vi "Import File - Tx XML.vi"(6 "Root Node":refnum<k24>, 8 "error in (no error)":errorcluster) -> (0 "error out":errorcluster, 5 "Tx Packets":T1 {"Tx Packet Data"."threadOptions"."pclDecimation" max=16 step=1; "Tx Packet Data"."threadOptions"."loopPeriod" max=16 step=1; "Tx Packet Data"."threadOptions"."targetPriority" min=-2 max=16 step=1; "Tx Packet Data"."threadOptions"."targetProcessor" min=-2 max=16 step=1; "Tx Packet Data"."Endianness" items=["big-endian"=0, "little-endian"=2]})   [LabVIEW 2019, in "UDP-Custom-Device System Explorer.lvlib"]
uses:
  UDP-Custom-Device System Explorer.lvlib
  System.Xml
  Types/XML - New/ImpExp - Tx Packets Data.ctl
  <vilib>/NI VeriStand/Custom Device API/Custom Device Item Info.ctl
  Types/XML - New/ImpExp - Tx Packet Data.ctl
  Shared/Types/Shared - Channel Data Type.ctl
  Shared/Types/Shared - Buffered.PacketInfo.ctl
  Shared/Types/Shared - Pointer Encoding.ctl
  Shared/Types/Shared - Receive Buffer Options.ctl
  Shared/Types/Shared - Transmit Buffer Options.ctl
  Shared/Types/Shared - Transmit Flag Options.ctl
  Shared/Types/Shared - Transmit Echo Options.ctl
  Types/Threading/Thread Configuration.ctl
  Types/Threading/Thread Sync Reference.ctl
  Shared/Types/Shared - Thread Management.ctl
  <vilib>/NI VeriStand/Custom Device API/Custom Device API.lvlib
  Shared/UDP-Custom-Device Shared.lvlib
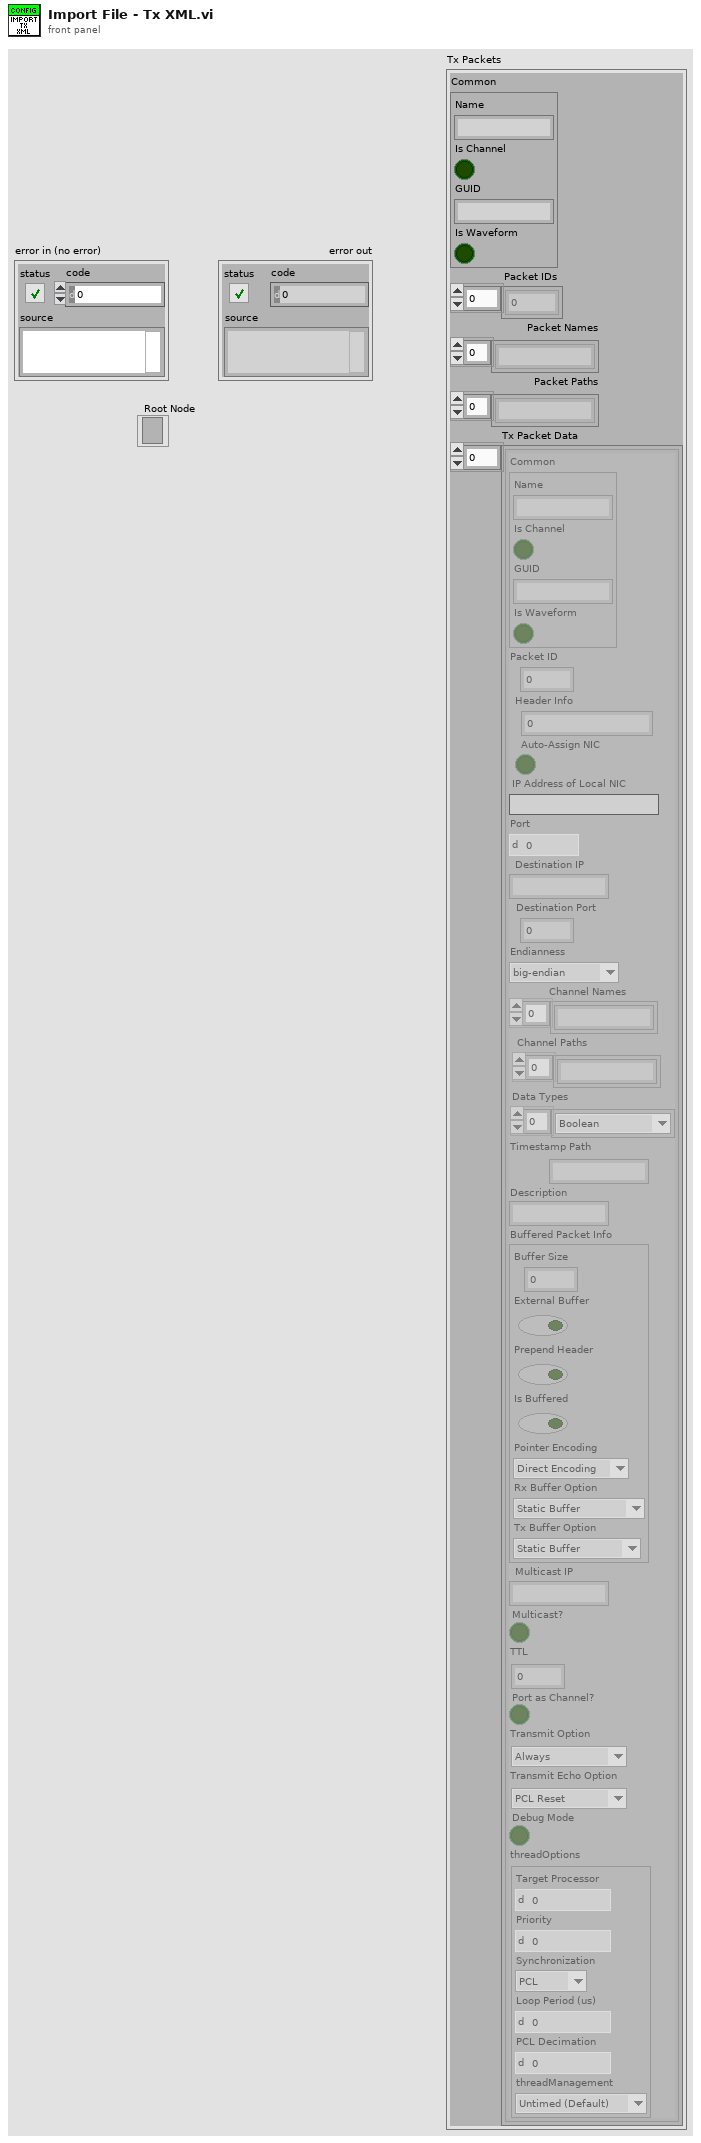
[diagram p1: front panel]
types:
  T1 = typedef "UDP-Custom-Device System Explorer.lvlib/ImpExp - Tx Packets Data.ctl" = cluster{"Common":T2, "Packet IDs":i32[], "Packet Names":string[], "Packet Paths":string[], "Tx Packet Data":T3[]}
  T2 = typedef "Custom Device API.lvlib/Custom Device Item Info.ctl" = cluster{"Name":string, "Is Channel":bool, "GUID":string, "Is Waveform":bool}
  T3 = typedef "UDP-Custom-Device System Explorer.lvlib/ImpExp - Tx Packet Data.ctl" = cluster{"Common":T2, "Packet ID":i32, "Header Info":u32, "Auto-Assign NIC":bool, "IP Address of Local NIC":string, "Port":u16, "Destination IP":string, "Destination Port":u16, "Endianness":u16, "Channel Names":string[], "Channel Paths":string[], "Data Types":T4[], "Timestamp Path":string, "Description":string, "Buffered Packet Info":T5, "Multicast IP":string, "Multicast?":bool, "TTL":u16, "Port as Channel?":bool, "Transmit Option":T9, "Transmit Echo Option":T10, "Debug Mode":bool, "threadOptions":T11}
  T4 = typedef "UDP-Custom-Device Shared.lvlib/Shared - Channel Data Type.ctl" = enum16{"Boolean", "Single", "Double", "I8", "I16", "I32", "I64", "U8", "U16", "U32", "U64"}
  T5 = typedef "UDP-Custom-Device Shared.lvlib/Shared - Buffered.PacketInfo.ctl" = cluster{"Buffer Size":i32, "External Buffer":bool, "Prepend Header":bool, "Is Buffered":bool, "Pointer Encoding":T6, "Rx Buffer Option":T7, "Tx Buffer Option":T8}
  T6 = typedef "UDP-Custom-Device Shared.lvlib/Shared - Pointer Encoding.ctl" = enum16{"Direct Encoding", "Conversion Encoding"}
  T7 = typedef "UDP-Custom-Device Shared.lvlib/Shared - Receive Buffer Options.ctl" = enum16{"Static Buffer", "Circular Buffer", "Circular Buffer + Size", "Internal Cache", "Internal Cache + Size", "Ping Pong", "Ping Pong + Size"}
  T8 = typedef "UDP-Custom-Device Shared.lvlib/Shared - Transmit Buffer Options.ctl" = enum16{"Static Buffer", "FIFO Buffer", "FIFO Buffer + Port"}
  T9 = typedef "UDP-Custom-Device Shared.lvlib/Shared - Transmit Flag Options.ctl" = enum16{"Always", "One-Shot", "Toggle"}
  T10 = typedef "UDP-Custom-Device Shared.lvlib/Shared - Transmit Echo Options.ctl" = enum16{"PCL Reset", "Counter", "Mirror"}
  T11 = typedef "UDP-Custom-Device System Explorer.lvlib/Thread Configuration.ctl" = cluster{"targetProcessor":i8, "targetPriority":i16, "Synchronization":T12, "loopPeriod":u32, "pclDecimation":u16, "threadManagement":T13}
  T12 = typedef "UDP-Custom-Device System Explorer.lvlib/Thread Sync Reference.ctl" = enum16{"PCL", "Async"}
  T13 = typedef "UDP-Custom-Device Shared.lvlib/Shared - Thread Management.ctl" = enum16{"Untimed (Default)", "Timed (High Priority)"}
  T14 = typedef "UDP-Custom-Device System Explorer.lvlib/ImpExp - Packet Headers.ctl" = cluster{"Packet Name":string, "Packet ID":string, "Packet Path":string}
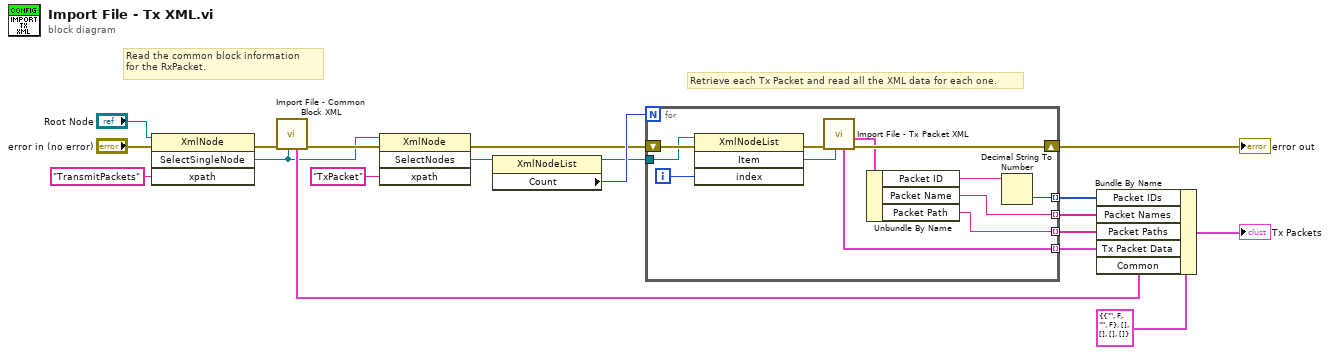
[diagram p0: block diagram]
diagram:
  # "Retrieve each Tx Packet and read all the XML data for each one."
  # "Read the common block information\nfor the RxPacket."
  n1 = invoke class="XmlNode" method="SelectSingleNode"(reference="Root Node", error in="error in (no error)", "xpath"="TransmitPackets") -> (error out=w19:errorcluster, "SelectSingleNode"=w9:refnum<k24>)  [unwired: 1 in, 2 out]
  n2 = call "Import File - Common Block XML.vi"("Root Node"=w9, "error in (no error)"=w19) -> ("error out"=w10:errorcluster, "Common"=w14:T2)  [unwired: 8 in]
  n3 = invoke class="XmlNode" method="SelectNodes"(reference=w9, error in=w10, "xpath"="TxPacket") -> (error out=w7:errorcluster, "SelectNodes"=w12:refnum<k24>)  [unwired: 1 in, 2 out]
  n4 = property class="XmlNodeList"(reference=w12) -> (reference out=w6:refnum<k24>, "Count"=w8:i32)  [unwired: 1 in, 1 out]
  n5 = for {
    N: w8 -> [_]
    shift-right: [w23] -> w5
    shift-left: w7 -> [w31]
    tunnel: w6 -> [w30]
    tunnel: [w27] -> w4 mode=indexing
    tunnel: [w26] -> w3 mode=indexing
    tunnel: [w25] -> w2 mode=indexing
    tunnel: [w21] -> w1 mode=indexing
    i -> [w29]
    n6 = invoke class="XmlNodeList" method="Item"(reference=w30, error in=w31, "index"=w29) -> (error out=w24:errorcluster, "Item"=w22:refnum<k24>)  [unwired: 1 in, 2 out]
    n7 = call "Import File - Tx Packet XML.vi"("Root Node"=w22, "error in (no error)"=w24) -> ("error out"=w23:errorcluster, "Packet Header Data"=w20:T14, "Tx Packet"=w21:T3)  [unwired: 7 in]
    n8 = Unbundle By Name(w20) -> ("Packet ID"=w28:string, "Packet Name"=w26:string, "Packet Path"=w25:string)
    n9 = Decimal String To Number(string=w28) -> (number=w27:i32)  [unwired: 2 in, 1 out]
  }
  "error out" <- w5
  n10 = Bundle By Name(cluster=T1 {"Common"={"Name"="", "Is Channel"=FALSE, "GUID"="", "Is Waveform"=FALSE}, "Packet IDs"=[], "Packet Names"=[], "Packet Paths"=[], "Tx Packet Data"=[]} ("Tx Packets"), "Packet IDs"=w4, "Packet Names"=w3, "Packet Paths"=w2, "Tx Packet Data"=w1, "Common"=w14) -> (→"Tx Packets":T1)
